vi "Main UI.vi"() -> ()   [LabVIEW 2016]
uses:
  Ctrls/Continuous Operations.ctl
  <vilib>/Utility/error.llb/DialogType.ctl
  HardWare/Ctrls/HardWare Gen _ DAQ Queue Names FGV Operations.ctl
  HardWare/Gantner/DAQ FGV Operations.ctl
  Architecture/Queue Management/ARC_Queue Create_Single.vi
  Architecture/Queue Management/ARC_Queue Valid.vi
  Architecture/Queue Management/ARC_Queue Remove Element.vi
  Ctrls/GlobeVaribles.vi
  Architecture/Queue Management/ARC_Queue Insert Element.vi
  Architecture/Queue Management/ARC_Queue Destroy_Single.vi
panel:
  in  "Tree":string(tree)
  in  "Stop":bool
  in  "Run":bool
  in  "Pause":bool
  out "notification":string
  out "变频器电压":sgl caption="Q1" format="%#.2f"
  out "变频器电流":sgl caption="Q2" format="%#.2f"
  out "变频器转速":sgl caption="Q3" format="%#.2f"
  out "变频器转矩":sgl caption="Q4" format="%#.2f"
  out "变频器加速时间":sgl caption="Q5" format="%#.2f"
  out "变频器减速时间":sgl caption="Q5" format="%#.2f"
  out "剩余时间":sgl caption="剩余时间:" format="%#.3g"
  out "设定时间":sgl caption="设定时间:" format="%#.3g"
  out "Error Report":string
  # "秒"
  # "秒"
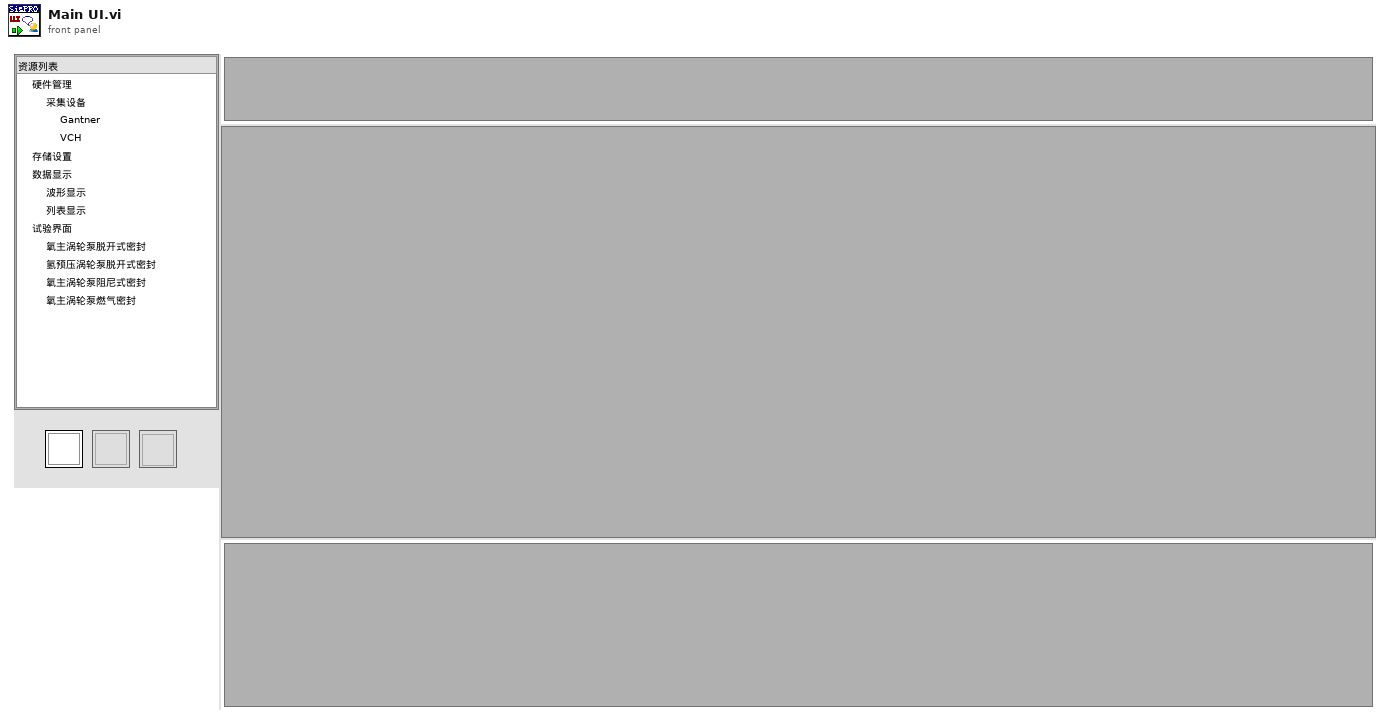
[diagram p1: front panel]
types:
  T1 = enum32{"Invalid", "Standard", "Closed", "Hidden", "Minimized", "Maximized"}
  T2 = enum16{"Obtain Notifier", "Send Notification", "Wait Notification", "Release Notifier"}
  T3 = typedef "Sys Paths.ctl" = cluster{"System Config":path, "User Archives":path, "Error Log":path, "DynaThreads":path, "TreePNG":path}
  T4 = typedef "User Login_Archives Data Structure.ctl" = cluster{"User Archives":cluster{"User Name":string, "Code":string, "Ability":enum16{"Administrator", "Operator"}, "Last Log Time":timestamp}[], "Current User":i32}
  T5 = cluster{"Error":errorcluster, "Exit":bool, "LocalQ":cluster{"LocalName":string, "LocalEvent":string, "LocalData":variant}, "Q-LowLevel":cluster{"Q-LowLevel Name":string, "Q-LowLevel Order":string, "Q-LowLevel Data":variant}, "Ref":cluster{"VIRef":refnum<vi>, "Tree":refnum<vi>}, "Threads":cluster{"Cfg":string, "Disp":string, "VCH":string, "Data":string, "SavePara":string}, "InsertUI":string, "Path":T3, "User Archives":T4, "FailedThreads":cluster{"ThreadName":string, "Fail":bool}[], "Buffers":cluster{"DataBuf":refnum<queue>}, "DevName":string}
  T6 = typedef "Continuous Operations.ctl" = enum16{"Writting", "Pause", "Stop"}
  T7 = typedef "HardWare Gen _ DAQ Queue Names FGV Operations.ctl" = enum16{"Initialize", "AddName", "ReadName"}
  T8 = typedef "DAQ FGV Operations.ctl" = enum16{"Search", "ReadCFG", "ReadVCH", "UpdateTempCFG", "DownloadCFG", "OpenCFG", "ImportPara", "Config", "Start", "Read", "Stop", "Clear"}
  T9 = typedef "DialogType.ctl" = u16
  T10 = cluster{"Run":refnum<vi>, "Pause":refnum<vi>, "Stop":refnum<vi>}
  T11 = cluster{"LocalName":string, "System Config":path, "DynaThreads":path, "DataBuf":refnum<queue>, "VIRef":refnum<vi>}
  T12 = cluster{"LocalName":string, "DataBuf":refnum<queue>}
  T13 = cluster{"LocalName":string, "System Config":path}
  T14 = typedef "LVRectTypeDef.ctl" = cluster{"Left":i16, "Top":i16, "Right":i16, "Bottom":i16}
  T15 = typedef "HardWare _ Module Configuration.ctl" = cluster{"ModuName":string, "ModuAlias":string, "ModuSN":string, "CHtype":string, "ParaNames[]":string[], "Paravalues[]":string[][]}
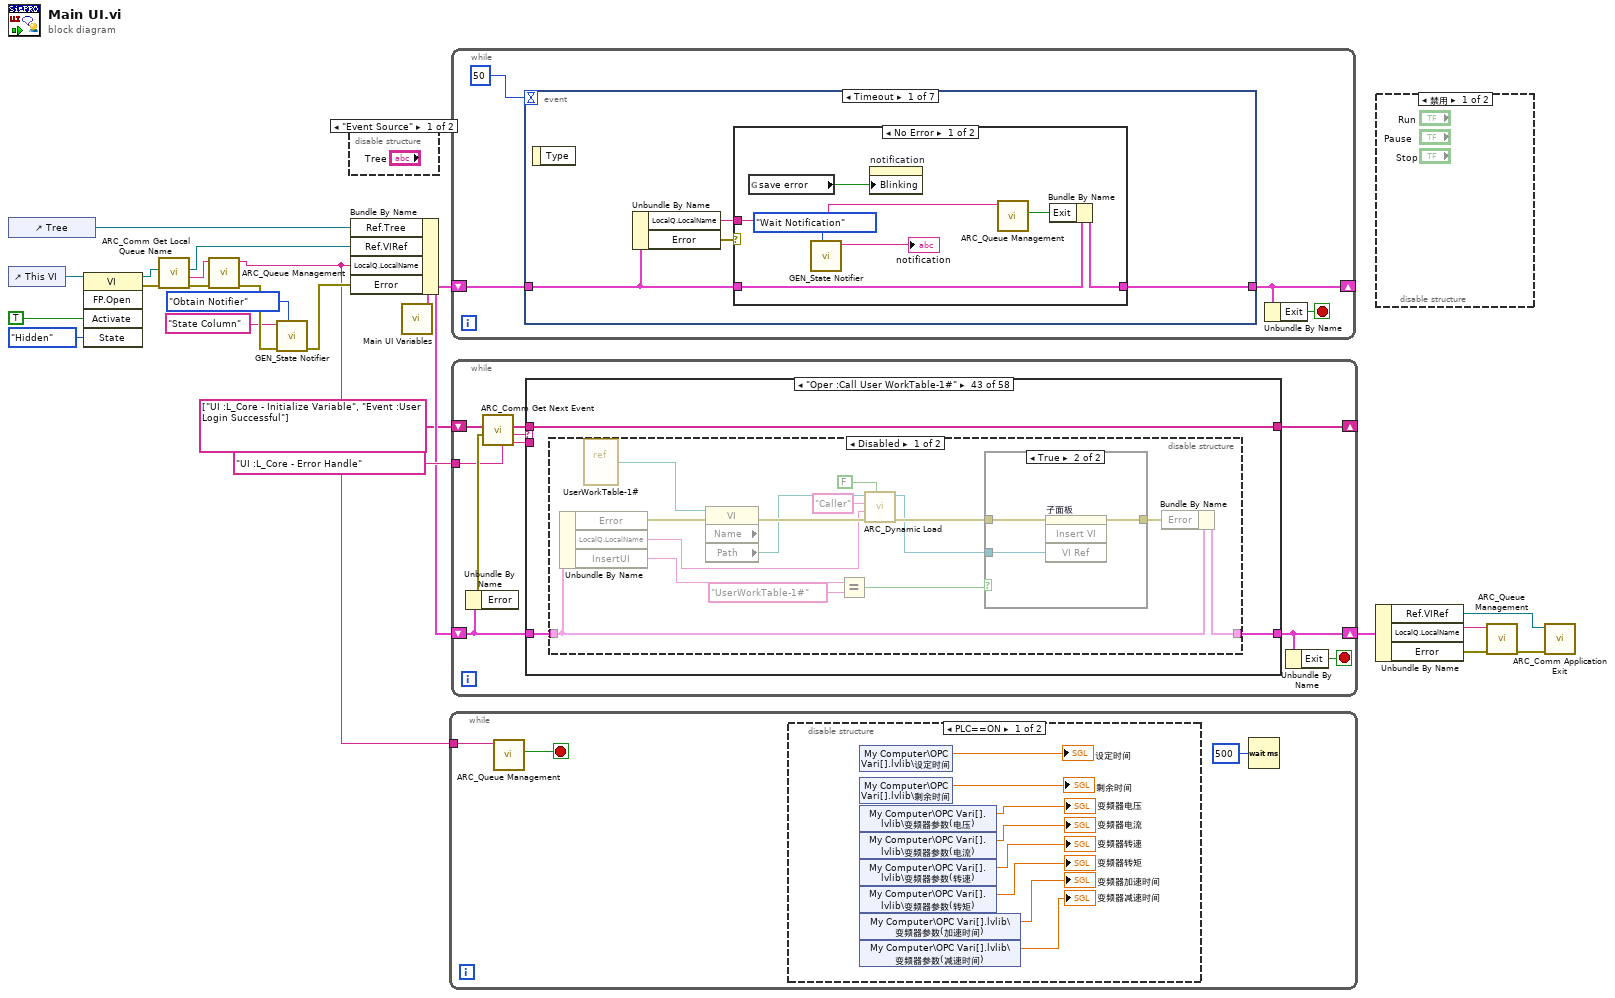
[diagram p0: block diagram]
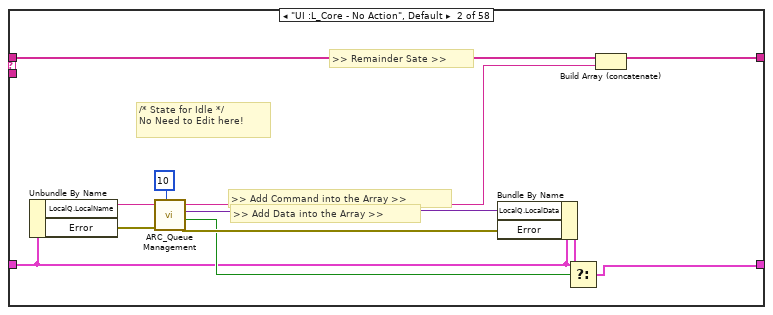
[diagram p6: hidden frame]
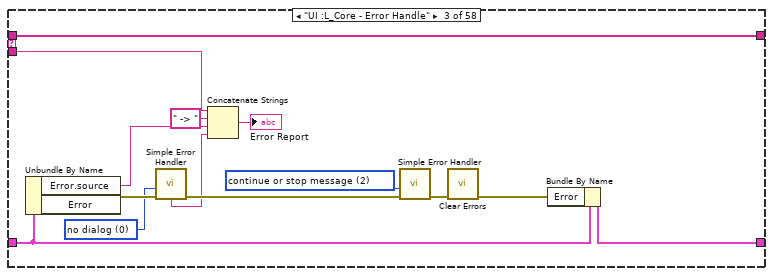
[diagram p7: hidden frame]
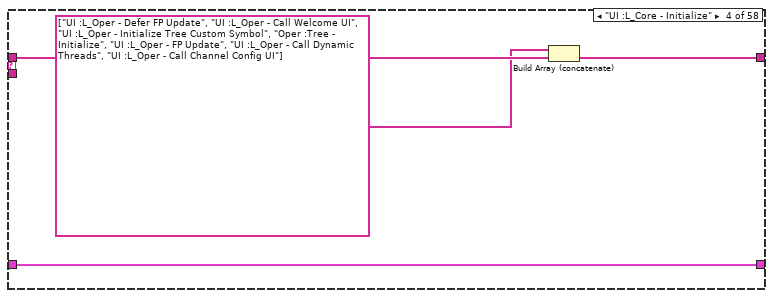
[diagram p8: hidden frame]
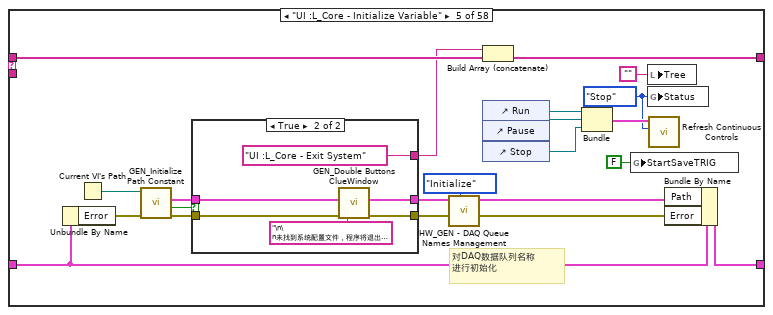
[diagram p9: hidden frame]
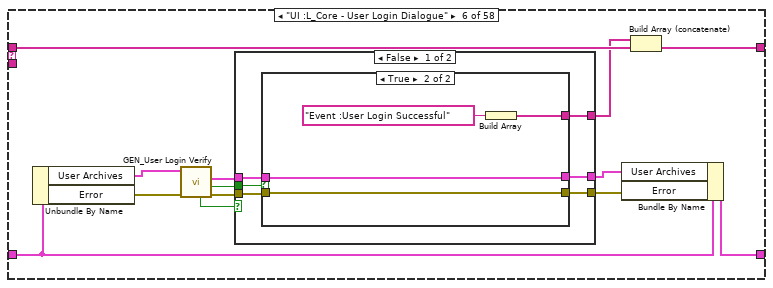
[diagram p11: hidden frame]
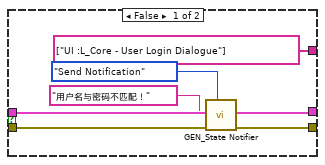
[diagram p12: hidden frame]
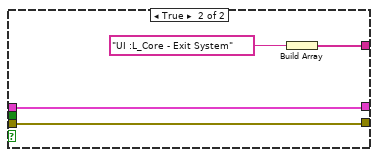
[diagram p13: hidden frame]
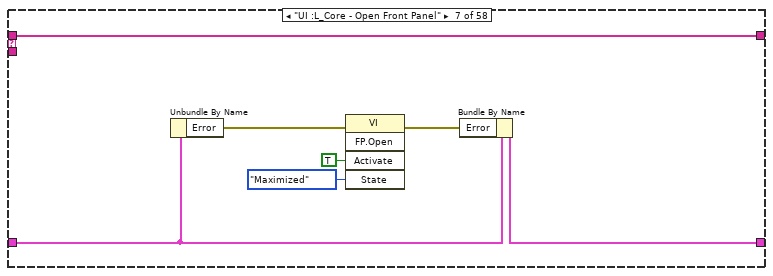
[diagram p14: hidden frame]
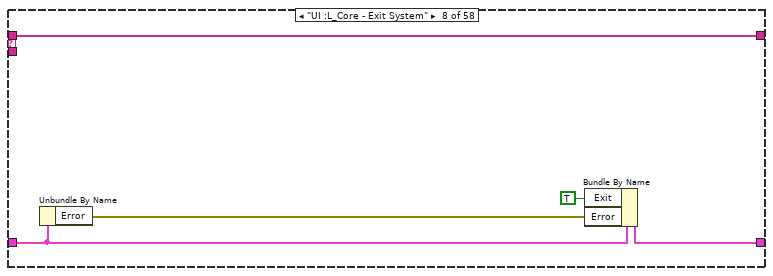
[diagram p15: hidden frame]
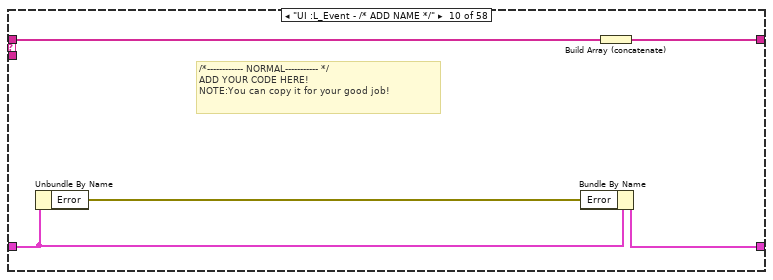
[diagram p17: hidden frame]
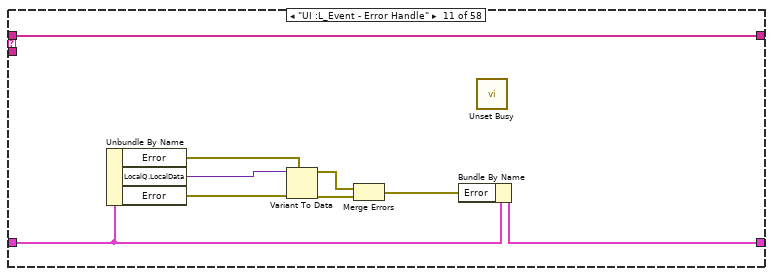
[diagram p18: hidden frame]
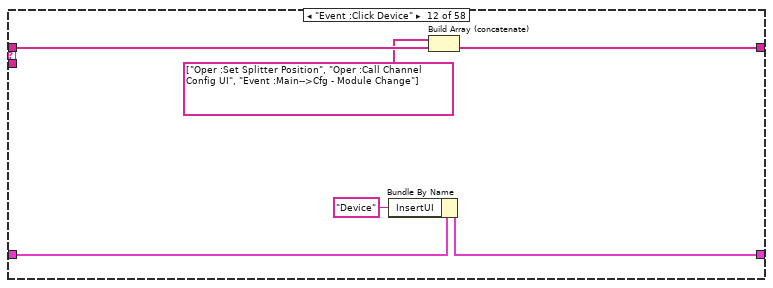
[diagram p19: hidden frame]
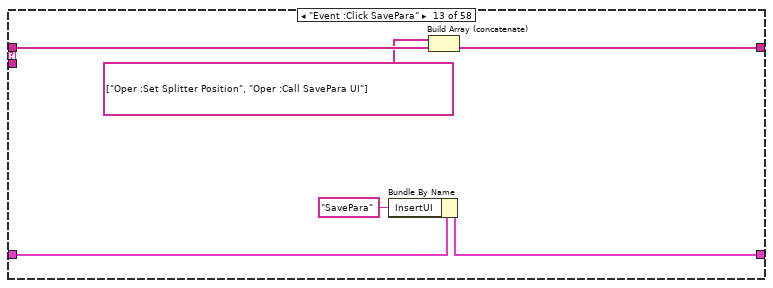
[diagram p20: hidden frame]
diagram:
  n1 = control-ref of="Tree"() -> (w15:refnum<vi>)
  n2 = control-ref of="This VI"() -> (w3:refnum<vi>)
  n3 = invoke class="VI" method="FP.Open"(reference=w3, "Activate"=TRUE ("激活？"), "State"=T1."Hidden" ("状态")) -> (reference out=w2:refnum<vi>, error out=w4:errorcluster)  [unwired: 2 in, 3 out]
  n4 = call "ARC_Comm Get Local Queue Name.vi"("error in"=w4, "VI Ref"=w2) -> ("error out"=w12:errorcluster, "VI  Name"=w14:string, "VI Ref out"=w13:refnum<vi>)  [unwired: 7 in]
  n5 = call-poly "ARC_Queue Management.vi"("error in"=w12, "Queue Name"=w14) -> ("error out"=w11:errorcluster, "Queue Name dup"=w1:string)  [unwired: 7 in, 1 out]
  n6 = call "GEN_State Notifier.vi"("Action Select"=T2."Obtain Notifier", "error in (no error)"=w11, "Notifier Name"="State Column") -> ("error out"=w10:errorcluster)  [unwired: 7 in, 1 out]
  n7 = disable-structure shown="\"Event Source\"" {
    frame condition #0 (active) {
    }
    frame condition #1 {
    }
  }
  n8 = call "Main UI Variables.vi"() -> ("Main UI.vi"=w16:T5)  [unwired: 11 in]
  n9 = Bundle By Name(cluster=w16, "Ref.Tree"=w15, "Ref.VIRef"=w13, "LocalQ.LocalName"=w1, "Error"=w10) -> (w20:T5)
  n10 = while {
    tunnel: w1 -> [w25]
    stop <- w24 stop-if-true
    n11 = call-poly "ARC_Queue Management.vi"("Queue Name(unamed)"=w25) -> ("Not Exist?"=w24:bool)  [unwired: 8 in, 2 out]
    n12 = disable-structure shown="PLC==ON" {
      frame condition #0 (active) {
        n13 = shared-variable "My Computer\\OPC Vari[].lvlib\\设定时间"() -> (→"设定时间":sgl)  [unwired: 1 in, 1 out]
        n14 = shared-variable "My Computer\\OPC Vari[].lvlib\\剩余时间"() -> (→"剩余时间":sgl)  [unwired: 1 in, 1 out]
        n15 = shared-variable "My Computer\\OPC Vari[].lvlib\\变频器参数(电压)"() -> (→"变频器电压":sgl)  [unwired: 1 in, 1 out]
        n16 = shared-variable "My Computer\\OPC Vari[].lvlib\\变频器参数(电流)"() -> (→"变频器电流":sgl)  [unwired: 1 in, 1 out]
        n17 = shared-variable "My Computer\\OPC Vari[].lvlib\\变频器参数(转速)"() -> (→"变频器转速":sgl)  [unwired: 1 in, 1 out]
        n18 = shared-variable "My Computer\\OPC Vari[].lvlib\\变频器参数(转矩)"() -> (→"变频器转矩":sgl)  [unwired: 1 in, 1 out]
        n19 = shared-variable "My Computer\\OPC Vari[].lvlib\\变频器参数(加速时间)"() -> (→"变频器加速时间":sgl)  [unwired: 1 in, 1 out]
        n20 = shared-variable "My Computer\\OPC Vari[].lvlib\\变频器参数(减速时间)"() -> (→"变频器减速时间":sgl)  [unwired: 1 in, 1 out]
      }
      frame condition #1 {
      }
    }
    n21 = Wait (ms)(milliseconds to wait=u32 500 ("等待时间（毫秒）")) -> ()  [unwired: 1 out]
  }
  n22 = while {
    shift-right: [w36] -> _
    shift-left: w20 -> [w37]
    stop <- w35 stop-if-true
    n23 = event shown="[0] Timeout" {
      selector: _ -> [_ _ _ _ _ _ _]
      dyn-events: _ -> [_ _ _ _ _ _ _]
      timeout: 50 -> [_ _ _ _ _ _ _]
      tunnel: w37 -> [w41 w61 w65 w79 w93 w113 w123]
      tunnel: [w42 w60 w64 w77 w92 w112 w122] -> w36
      event Timeout {
        n24 = event-data() -> ()  [unwired: 1 in, 1 out]
        n25 = Unbundle By Name(w41) -> ("LocalQ.LocalName"=w40:string, "Error"=w39:errorcluster)
        n26 = case shown="No Error" w39 {
          selector: w39 -> [_ w56]
          tunnel: [w49 w54] -> w42
          tunnel: w41 -> [w47 w55]
          tunnel: w40 -> [w46 w53]
          frame No Error {
            n27 = global read "GlobeVaribles.vi" "save error"() -> (w44:bool)
            n28 = call "GEN_State Notifier.vi"("Action Select"=T2."Wait Notification") -> ("Notification out"=→"notification":string)  [unwired: 9 in, 1 out]
            n29 = property on="notification" class="Str"("Blinking"=w44) -> ()  [unwired: 2 in, 2 out]
            n30 = call-poly "ARC_Queue Management.vi"("Queue Name(unamed)"=w46) -> ("Not Exist?"=w48:bool)  [unwired: 8 in, 2 out]
            n31 = Bundle By Name(cluster=w47, "Exit"=w48) -> (w49:T5)
          }
          frame Error {
            n32 = To Variant(anything=w56) -> (Variant=w51:variant)
            n33 = call "ARC_Queue Insert Single Messenges.vi"("Data"=w51, "Order"="UI :L_Event - Error Handle" ("Event"), "Queue Name"=w53) -> ("error out"=w50:errorcluster)  [unwired: 8 in]
            n34 = Bundle By Name(cluster=w55, "Error"=w50) -> (w54:T5)
          }
        }
      }
      event Panel Close? {
        n35 = event-data() -> ()  [unwired: 1 in, 1 out]
        n36 = Unbundle By Name(w61) -> ("LocalQ.LocalName"=w58:string, "Error"=w62:errorcluster)
        n37 = call-poly "ARC_Queue Management.vi"("error in (no error)"=w62, "Event"="UI :L_Event - Exit Event", "Queue Name(unamed)"=w58) -> ("error out"=w59:errorcluster)  [unwired: 7 in, 1 out]
        n38 = Bundle By Name(cluster=w61, "Error"=w59) -> (w60:T5)
        n39 = event-data("Discard?"=TRUE ("放弃？")) -> ()  [unwired: 1 in, 1 out]
      }
      event Panel Resize {
        n40 = event-data() -> ()  [unwired: 1 in, 1 out]
        n41 = Unbundle By Name(w65) -> ("LocalQ.LocalName"=w66:string, "Error"=w68:errorcluster)
        n42 = call-poly "ARC_Queue Management.vi"("error in (no error)"=w68, "Event"="Oper :Set Splitter Position", "Queue Name(unamed)"=w66) -> ("error out"=w67:errorcluster)  [unwired: 7 in, 1 out]
        n43 = Bundle By Name(cluster=w65, "Error"=w67) -> (w64:T5)
      }
      event "Tree": Value Change {
        n44 = event-data() -> ("CtlRef"=w80:refnum<vi>, "NewVal"=w70:string)  [unwired: 1 in]
        n45 = Unbundle By Name(w79) -> ("Error"=w78:errorcluster, "LocalQ.LocalName"=w72:string)
        n46 = call "Main Tree _ Click Event Pharse(tag).vi"("error in"=w78, "tag in"=w70, "Ref.Tree Ref"=w80) -> ("error out"=w75:errorcluster, "cmd?"=w76:bool, "LocalData"=w74:variant, "LocalEvent"=w73:string)  [unwired: 5 in]
        n47 = case shown="True" w76 {
          tunnel: w75 -> [w81 w87]
          tunnel: w74 -> [_ w86]
          tunnel: w73 -> [_ w84]
          tunnel: w72 -> [_ w85]
          tunnel: [w81 w83] -> w71
          frame False {
          }
          frame True {
            n48 = call-poly "ARC_Queue Management.vi"("Time out(-1)_queue in"=20, "error in (no error)"=w87, "Data"=w86, "Event"=w84, "Queue Name(unamed)"=w85) -> ("error out"=w83:errorcluster)  [unwired: 5 in, 1 out]
          }
        }
        n49 = Bundle By Name(cluster=w79, "Error"=w71) -> (w77:T5)
      }
      event "Run": Value Change {
        n50 = event-data() -> ("CtlRef"=w94:refnum<vi>)  [unwired: 1 in]
        n51 = Unbundle By Name(w93) -> ("LocalQ.LocalName"=w91:string, "Error"=w95:errorcluster)
        n52 = invoke class="Bool" method="Reinit To Default"(reference=w94, error in=w95) -> (error out=w96:errorcluster)  [unwired: 1 in, 2 out]
        n53 = global read "GlobeVaribles.vi" "Status"() -> (w90:T6)
        n54 = case shown="\"Stop\"" w90 {
          tunnel: w96 -> [w100 w102 w107]
          tunnel: [w100 w102 w105] -> w89
          tunnel: w91 -> [_ _ w103]
          frame "Writting" {
          }
          frame "Pause", Default {
            n55 = global write "GlobeVaribles.vi" "Status"(Continuous_Operations."Writting" ("Status")) -> ()
          }
          frame "Stop" {
            n56 = call-poly "ARC_Queue Management.vi"("Time out(-1)_queue in"=50, "error in (no error)"=w107, "Event"="Event :Start Save", "Queue Name(unamed)"=w103) -> ("error out"=w105:errorcluster)  [unwired: 6 in, 1 out]
          }
        }
        n57 = flat-sequence {
          tunnel: w89 -> [w98]
          tunnel: [w97] -> w88
          frame #0 {
            n58 = call "Refresh Continuous Controls.vi"("error in"=w98, "Cmd"=Continuous_Operations."Writting") -> ("error out"=w97:errorcluster)  [unwired: 9 in]
          }
        }
        n59 = Bundle By Name(cluster=w93, "Error"=w88) -> (w92:T5)
      }
      event "Pause": Value Change {
        w108 = Continuous_Operations."Pause" ("Cmd")
        n60 = event-data() -> ("CtlRef"=w114:refnum<vi>)  [unwired: 1 in]
        n61 = Unbundle By Name(w113) -> ("LocalQ.LocalName"=w109:string, "Error"=w115:errorcluster)
        n62 = invoke class="Bool" method="Reinit To Default"(reference=w114, error in=w115) -> (error out=w117:errorcluster)  [unwired: 1 in, 2 out]
        n63 = call-poly "ARC_Queue Management.vi"("Time out(-1)_queue in"=50, "error in (no error)"=w117, "Event"="Event :Pause Save", "Queue Name(unamed)"=w109) -> ("error out"=w111:errorcluster)  [unwired: 6 in, 1 out]
        n64 = call "Refresh Continuous Controls.vi"("Cmd"=w108) -> ()  [unwired: 10 in, 1 out]
        n65 = global write "GlobeVaribles.vi" "Status"(w108) -> ()
        n66 = Bundle By Name(cluster=w113, "Error"=w111) -> (w112:T5)
      }
      event "Stop": Value Change {
        w118 = Continuous_Operations."Stop" ("Cmd")
        n67 = event-data() -> ("CtlRef"=w124:refnum<vi>)  [unwired: 1 in]
        n68 = Unbundle By Name(w123) -> ("LocalQ.LocalName"=w119:string, "Error"=w125:errorcluster)
        n69 = invoke class="Bool" method="Reinit To Default"(reference=w124, error in=w125) -> (error out=w127:errorcluster)  [unwired: 1 in, 2 out]
        n70 = call-poly "ARC_Queue Management.vi"("Time out(-1)_queue in"=50, "error in (no error)"=w127, "Event"="Event :Stop Save", "Queue Name(unamed)"=w119) -> ("error out"=w121:errorcluster)  [unwired: 6 in, 1 out]
        n71 = call "Refresh Continuous Controls.vi"("Cmd"=w118) -> ()  [unwired: 10 in, 1 out]
        n72 = global write "GlobeVaribles.vi" "Status"(w118) -> ()
        n73 = Bundle By Name(cluster=w123, "Error"=w121) -> (w122:T5)
      }
    }
    n74 = Unbundle By Name(w36) -> ("Exit"=w35:bool)
  }
  n75 = while {
    shift-right: [w131] -> w17
    shift-left: w20 -> [w133]
    shift-right: [w134] -> _
    shift-left: string[] ["UI :L_Core - Initialize Variable", "Event :User Login Successful"] ("event queue out") -> [w137]
    tunnel: "UI :L_Core - Error Handle" ("Error Handle") -> [w129]
    stop <- w130 stop-if-true
    n76 = Unbundle By Name(w133) -> ("Error"=w132:errorcluster)
    n77 = call "ARC_Comm Get Next Event.vi"("Error Handle"=w129, "error in (no error)"=w132, "event queue in"=w137) -> ("prev event"=w128:string, "next event"=w136:string, "event queue out"=w135:string[])  [unwired: 3 in]
    n78 = case shown="\"Oper :Call User WorkTable-1#\"" w136 {
      selector: w136 -> [_ _ _ _ _ _ _ _ _ _ _ _ _ _ _ _ _ _ _ _ _ _ _ _ _ w319 w328 w337 w346 w355 w366 w375 w386 _ _ _ _ _ _ _ _ _ _ _ _ _ _ _ _ _ _ _ _ _ _ _ _ _]
      tunnel: w133 -> [w138 w142 w163 w166 w186 w209 w232 w239 w243 w248 w251 w263 w269 w275 w281 w287 w293 w295 w297 w301 w303 w307 w309 w313 w317 w326 w335 w344 w353 w362 w372 w381 w392 w394 w401 w424 w465 w506 w547 w576 w604 w617 w628 w659 w681 w702 w725 w731 w735 w746 w757 w759 w770 w782 w790 w799 w801 w803]
      tunnel: w135 -> [w139 w148 w165 w169 w190 w210 w237 w242 w244 w246 w258 w264 w270 w276 w282 w288 w291 w296 w298 w302 w306 w308 w312 w316 w318 w327 w336 w345 w354 w363 w373 w382 w393 w395 w404 w429 w470 w511 w552 w583 w610 w622 w629 w665 w682 w703 w726 w732 w743 w754 w758 w761 w771 w783 w791 w800 w802 w811]
      tunnel: [w139 w147 w165 w168 w183 w202 w237 w242 w244 w245 w258 w262 w268 w274 w280 w286 w290 w296 w298 w300 w305 w308 w311 w315 w318 w324 w333 w342 w351 w360 w373 w382 w393 w395 w399 w429 w470 w511 w552 w583 w610 w622 w629 w665 w677 w703 w726 w732 w743 w754 w758 w761 w771 w779 w791 w800 w802 w811] -> w134
      tunnel: [w138 w140 w164 w166 w188 w200 w231 w240 w243 w247 w250 w260 w266 w272 w278 w284 w292 w295 w297 w301 w303 w307 w309 w313 w317 w325 w334 w343 w352 w361 w368 w377 w388 w394 w397 w423 w464 w505 w546 w575 w603 w616 w627 w658 w675 w695 w724 w730 w734 w745 w757 w759 w767 w780 w786 w794 w801 w810] -> w131
      tunnel: w128 -> [_ _ w153 _ _ _ _ _ _ _ _ _ _ _ _ _ _ _ _ _ _ _ _ _ _ _ _ _ _ _ _ _ _ _ _ _ _ _ _ _ _ _ _ _ _ _ _ _ _ _ _ _ _ _ _ _ _ _]
      frame "----------Core Status----------" {
      }
      frame "UI :L_Core - No Action", Default {
        # "/* State for Idle */\nNo Need to Edit here!"
        # ">> Add Data into the Array >>"
        # ">> Add Command into the Array >>"
        # ">> Remainder Sate >>"
        n79 = Unbundle By Name(w142) -> ("LocalQ.LocalName"=w145:string, "Error"=w149:errorcluster)
        n80 = call-poly "ARC_Queue Management.vi"("Time out(-1)_queue out"=10, "error in (no error)"=w149, "Queue Name(unamed)"=w145) -> ("error out"=w151:errorcluster, "timed out"=w143:bool, "Data"=w150:variant, "Event"=w146:string)  [unwired: 5 in]
        n81 = Bundle By Name(cluster=w142, "LocalQ.LocalData"=w150, "Error"=w151) -> (w141:T5)
        n82 = Select(t=w142, s=w143, f=w141) -> (s? t:f=w140:T5)
        n83 = Build Array (concatenate)(w148, w146) -> (w147:string[])
      }
      frame "UI :L_Core - Error Handle" {
        w152 = T9 0 items=["no dialog", "OK message", "continue or stop message", "OK message + warnings", "continue/stop + warnings"] ("type of dialog (OK msg:1)")
        w160 = T9 2 items=["no dialog", "OK message", "continue or stop message", "OK message + warnings", "continue/stop + warnings"] ("type of dialog (OK msg:1)")
        n84 = Unbundle By Name(w163) -> ("Error.source"=w154:string, "Error"=w157:errorcluster)
        n85 = call <vilib>:"Simple Error Handler.vi"("type of dialog (OK msg:1)"=w152, "error in (no error)"=w157) -> ("error out"=w156:errorcluster, "message"=w155:string)  [unwired: 3 in, 3 out]
        n86 = Concatenate Strings(w153, " -> " ("字符串"), w154, w155) -> (→"Error Report":string)
        n87 = call <vilib>:"Simple Error Handler.vi"("type of dialog (OK msg:1)"=w160, "error in (no error)"=w156) -> ("error out"=w162:errorcluster)  [unwired: 3 in, 4 out]
        n88 = call <vilib>:"Clear Errors.vi"("error in (no error)"=w162) -> ("error out"=w161:errorcluster)  [unwired: 5 in, 1 out]
        n89 = Bundle By Name(cluster=w163, "Error"=w161) -> (w164:T5)
      }
      frame "UI :L_Core - Initialize" {
        n90 = Build Array (concatenate)(string[] ["UI :L_Oper - Defer FP Update", "UI :L_Oper - Call Welcome UI", "UI :L_Oper - Initialize Tree Custom Symbol", "Oper :Tree - Initialize", "UI :L_Oper - FP Update", "UI :L_Oper - Call Dynamic Threads", "UI :L_Oper - Call Channel Config UI"], w169) -> (w168:string[])
      }
      frame "UI :L_Core - Initialize Variable" {
        w174 = Continuous_Operations."Stop" ("Status")
        # "对DAQ数据队列名称\n进行初始化"
        n91 = Unbundle By Name(w186) -> ("Error"=w185:errorcluster)
        n92 = Current VI's Path() -> (path=w187:path)
        n93 = call "GEN_Initialize Path Constant.vi"("error in"=w185, "Path in"=w187) -> ("error out"=w184:errorcluster, "File not exists?"=w181:bool, "Path Constant"=w180:T3)  [unwired: 6 in, 1 out]
        n94 = case shown="True" w181 {
          tunnel: w184 -> [w192 w195]
          tunnel: [w192 w194] -> w178
          tunnel: w180 -> [w191 w197]
          tunnel: [w191 w197] -> w179
          tunnel: [_ "UI :L_Core - Exit System"] -> w182
          frame False {
          }
          frame True {
            n95 = call "GEN_Double Buttons ClueWindow.vi"("error in (no error)"=w195, "Content Input"="\n\n未找到系统配置文件，程序将退出！" ("消息")) -> ("error out"=w194:errorcluster)  [unwired: 7 in, 2 out]
          }
        }
        n96 = call "HW_GEN - DAQ Queue Names Management.vi"("Oper."=HardWare_Gen___DAQ_Queue_Names_FGV_Operations."Initialize", "error in"=w178) -> ("error out"=w177:errorcluster)  [unwired: 8 in, 1 out]
        n97 = Build Array (concatenate)(w182, w190) -> (w183:string[])
        n98 = control-ref of="Run"() -> (w173:refnum<vi>)
        n99 = control-ref of="Pause"() -> (w172:refnum<vi>)
        n100 = control-ref of="Stop"() -> (w171:refnum<vi>)
        n101 = Bundle("Run"=w173, "Pause"=w172, "Stop"=w171) -> (w175:T10)  [unwired: 1 in]
        n102 = global write "GlobeVaribles.vi" "StartSaveTRIG"(FALSE ("StartSaveTRIG")) -> ()
        n103 = local write "Tree"("") -> ()
        n104 = global write "GlobeVaribles.vi" "Status"(w174) -> ()
        n105 = call "Refresh Continuous Controls.vi"("Cmd"=w174, "Ctrls"=w175) -> ()  [unwired: 9 in, 1 out]
        n106 = Bundle By Name(cluster=w186, "Path"=w179, "Error"=w177) -> (w188:T5)
      }
      frame "UI :L_Core - User Login Dialogue" {
        n107 = Unbundle By Name(w209) -> ("User Archives"=w208:T4, "Error"=w207:errorcluster)
        n108 = call "GEN_User Login Verify.vi"("error in"=w207, "User Archives"=w208) -> ("error out"=w206:errorcluster, "User Exist?"=w203:bool, "User Archives out"=w204:T4, "Cancel?"=w205:bool)  [unwired: 6 in]
        n109 = case shown="False" w205 {
          tunnel: w203 -> [w216 _]
          tunnel: w206 -> [w215 w228]
          tunnel: w204 -> [w214 w227]
          tunnel: [w213 w228] -> w199
          tunnel: [w212 w227] -> w198
          tunnel: [w211 w229] -> w201
          frame False {
            n110 = case shown="True" w216 {
              tunnel: w215 -> [w218 w226]
              tunnel: w214 -> [w222 w225]
              tunnel: [w222 w225] -> w212
              tunnel: [w219 w226] -> w213
              tunnel: [string[] ["UI :L_Core - User Login Dialogue"] w223] -> w211
              frame False {
                n111 = call "GEN_State Notifier.vi"("Action Select"=T2."Send Notification", "error in (no error)"=w218, "Notification"="用户名与密码不匹配！") -> ("error out"=w219:errorcluster)  [unwired: 7 in, 1 out]
              }
              frame True {
                n112 = Build Array("Event :User Login Successful") -> (w223:string[])
              }
            }
          }
          frame True {
            n113 = Build Array("UI :L_Core - Exit System") -> (w229:string[])
          }
        }
        n114 = Bundle By Name(cluster=w209, "User Archives"=w198, "Error"=w199) -> (w200:T5)
        n115 = Build Array (concatenate)(w201, w210) -> (w202:string[])
      }
      frame "UI :L_Core - Open Front Panel" {
        n116 = Unbundle By Name(w232) -> ("Error"=w235:errorcluster)
        n117 = invoke class="VI" method="FP.Open"(error in=w235, "Activate"=TRUE ("激活？"), "State"=T1."Maximized" ("状态")) -> (error out=w236:errorcluster)  [unwired: 2 in, 4 out]
        n118 = Bundle By Name(cluster=w232, "Error"=w236) -> (w231:T5)
      }
      frame "UI :L_Core - Exit System" {
        n119 = Unbundle By Name(w239) -> ("Error"=w241:errorcluster)
        n120 = Bundle By Name(cluster=w239, "Exit"=TRUE, "Error"=w241) -> (w240:T5)
      }
      frame "----------Events----------" {
        # ">> Notes: 此处分支主要用于响应事件结构，考虑多个事件的合并，可在此处执行代码后进行界面刷新；<<"
      }
      frame "UI :L_Event - /* ADD NAME */" {
        # "/*------------ NORMAL----------- */\nADD YOUR CODE HERE!\nNOTE:You can copy it for your good job!"
        n121 = Unbundle By Name(w248) -> ("Error"=w249:errorcluster)
        n122 = Bundle By Name(cluster=w248, "Error"=w249) -> (w247:T5)
        n123 = Build Array (concatenate)(w246) -> (w245:string[])
      }
      frame "UI :L_Event - Error Handle" {
        n124 = Unbundle By Name(w251) -> ("Error"=w255:errorcluster, "LocalQ.LocalData"=w256:variant, "Error"=w257:errorcluster)
        n125 = Variant To Data(error in=w257, type=w255, Variant=w256) -> (data=w254:errorcluster, error out=w252:errorcluster)
        n126 = Merge Errors(w254, w252) -> (w253:errorcluster)
        n127 = Bundle By Name(cluster=w251, "Error"=w253) -> (w250:T5)
        n128 = call <vilib>:"Unset Busy.vi"() -> ()  [unwired: 11 in, 1 out]
      }
      frame "Event :Click Device" {
        n129 = Bundle By Name(cluster=w263, "InsertUI"="Device") -> (w260:T5)
        n130 = Build Array (concatenate)(string[] ["Oper :Set Splitter Position", "Oper :Call Channel Config UI", "Event :Main-->Cfg - Module Change"] ("数组"), w264) -> (w262:string[])
      }
      frame "Event :Click SavePara" {
        n131 = Bundle By Name(cluster=w269, "InsertUI"="SavePara") -> (w266:T5)
        n132 = Build Array (concatenate)(string[] ["Oper :Set Splitter Position", "Oper :Call SavePara UI"] ("数组"), w270) -> (w268:string[])
      }
      frame "Event :Click Graph" {
        # "//单击波形图显示界面"
        n133 = Bundle By Name(cluster=w275, "InsertUI"="Q_Disp") -> (w272:T5)
        n134 = Build Array (concatenate)(string[] ["Oper :Set Splitter Position", "Oper :Call Display Graph", "Event :Main-->Disp - Graph UI"] ("数组"), w276) -> (w274:string[])
      }
      frame "Event :Click List" {
        # "//单击列表显示界面"
        n135 = Bundle By Name(cluster=w281, "InsertUI"="Q_Disp") -> (w278:T5)
        n136 = Build Array (concatenate)(string[] ["Oper :Set Splitter Position", "Oper :Call Display Graph", "Event :Main-->Disp - List UI"] ("数组"), w282) -> (w280:string[])
      }
      frame "Event :Click UserWorkTable-1#" {
        n137 = Bundle By Name(cluster=w287, "InsertUI"="UserWorkTable-1#") -> (w284:T5)
        n138 = Build Array (concatenate)(string[] ["Oper :Set Splitter Position", "Oper :Call User WorkTable-1#", "Event :Main-->Disp - List UI"] ("数组"), w288) -> (w286:string[])
      }
      frame "UI :L_Event - Exit Event" {
        n139 = Unbundle By Name(w293) -> ("Error"=w294:errorcluster)
        n140 = Bundle By Name(cluster=w293, "Error"=w294) -> (w292:T5)
        n141 = Build Array (concatenate)(w291, string[] ["UI :L_Core - Exit System"] ("数组")) -> (w290:string[])
      }
      frame "----------events from other threads----------" {
      }
      frame "Event :Error Handle" {
      }
      frame "Event :User Login Successful" {
        n142 = Build Array (concatenate)(string[] ["UI :L_Oper - Defer FP Update", "UI :L_Oper - Set Mouse Busy", "UI :L_Oper - Initialize Tree Custom Symbol", "Oper :Tree - Initialize", "Oper :Set Splitter Position", "Oper :Set User Group Menus", "UI :L_Oper - FP Update", "Oper :Create Buffers", "Oper :Call Dynamic Threads", "Oper :Scan for Devices", "UI :L_Oper - Set Mouse Free"], w302) -> (w300:string[])
      }
      frame "Event :Cfg-->M - Update ChanPara" {
        # "//接收配置线程发送过来的设备参数信息修改命令"
        n143 = Build Array (concatenate)(string[] ["Event :Main-->Disp - Update Channel Para", "Event :Main-->Data - Update Channel Para"] ("数组"), w306) -> (w305:string[])
      }
      frame "Event :Cfg-->M - Unbusy Mouse" {
        n144 = call <vilib>:"Unset Busy.vi"() -> ()  [unwired: 11 in, 1 out]
      }
      frame "Event :Start Save" {
        # "主线程收到显示线程的命令，启动连续存储；\n主线程向数据线程发送命令；"
        n145 = Build Array (concatenate)("Event :Main-->Data - Start Save", w312) -> (w311:string[])
      }
      frame "Event :Stop Save" {
        # "主线程收到显示线程的命令，停止连续存储；\n主线程向数据线程发送命令；"
        n146 = Build Array (concatenate)("Event :Main-->Data - Stop Save", w316) -> (w315:string[])
      }
      frame "---------------send to other threads--------------" {
      }
      frame "Event :Main-->Cfg - Module Change" {
        # "//单击tree上某模块名称后，向配置线程发送选择的模块信息"
        n147 = Unbundle By Name(w326) -> ("Threads.Cfg"=w322:string, "LocalQ.LocalData"=w320:variant, "Error"=w321:errorcluster)
        n148 = Bundle By Name(cluster=w326, "Q-LowLevel.Q-LowLevel Order"=w319, "Q-LowLevel.Q-LowLevel Name"=w322, "Q-LowLevel.Q-LowLevel Data"=w320, "Error"=w321) -> (w325:T5)
        n149 = Build Array (concatenate)("Oper :Send To LowLevel" ("Error Handle"), w327) -> (w324:string[])
        n150 = call <vilib>:"Set Busy.vi"() -> ()  [unwired: 10 in, 2 out]
      }
      frame "Event :Main-->Cfg - Start DAQ" {
        # "//单击tree上某模块名称后，向配置线程发送选择的模块信息"
        n151 = Unbundle By Name(w335) -> ("Threads.Cfg"=w331:string, "LocalQ.LocalData"=w329:variant, "Error"=w330:errorcluster)
        n152 = Bundle By Name(cluster=w335, "Q-LowLevel.Q-LowLevel Order"=w328, "Q-LowLevel.Q-LowLevel Name"=w331, "Q-LowLevel.Q-LowLevel Data"=w329, "Error"=w330) -> (w334:T5)
        n153 = Build Array (concatenate)("Oper :Send To LowLevel" ("Error Handle"), w336) -> (w333:string[])
      }
      frame "Event :Main-->Disp - Update Channel Para" {
        n154 = Unbundle By Name(w344) -> ("Threads.Disp"=w340:string, "LocalQ.LocalData"=w338:variant, "Error"=w339:errorcluster)
        n155 = Bundle By Name(cluster=w344, "Q-LowLevel.Q-LowLevel Order"=w337, "Q-LowLevel.Q-LowLevel Name"=w340, "Q-LowLevel.Q-LowLevel Data"=w338, "Error"=w339) -> (w343:T5)
        n156 = Build Array (concatenate)("Oper :Send To LowLevel" ("Error Handle"), w345) -> (w342:string[])
      }
      frame "Event :Main-->Disp - Graph UI" {
        n157 = Unbundle By Name(w353) -> ("Threads.Disp"=w349:string, "LocalQ.LocalData"=w347:variant, "Error"=w348:errorcluster)
        n158 = Bundle By Name(cluster=w353, "Q-LowLevel.Q-LowLevel Order"=w346, "Q-LowLevel.Q-LowLevel Name"=w349, "Q-LowLevel.Q-LowLevel Data"=w347, "Error"=w348) -> (w352:T5)
        n159 = Build Array (concatenate)("Oper :Send To LowLevel" ("Error Handle"), w354) -> (w351:string[])
      }
      frame "Event :Main-->Disp - List UI" {
        n160 = Unbundle By Name(w362) -> ("Threads.Disp"=w358:string, "LocalQ.LocalData"=w356:variant, "Error"=w357:errorcluster)
        n161 = Bundle By Name(cluster=w362, "Q-LowLevel.Q-LowLevel Order"=w355, "Q-LowLevel.Q-LowLevel Name"=w358, "Q-LowLevel.Q-LowLevel Data"=w356, "Error"=w357) -> (w361:T5)
        n162 = Build Array (concatenate)("Oper :Send To LowLevel" ("Error Handle"), w363) -> (w360:string[])
      }
      frame "Event :Main-->Data - Start Save" {
        # "给启动存储的触发信号\n让DAQ线程建立时间通道信息"
        # "主线程收到显示线程的命令，启动连续存储；\n主线程向数据线程发送命令；"
        n163 = Unbundle By Name(w372) -> ("Threads.Data"=w370:string, "Error"=w371:errorcluster)
        n164 = call-poly "ARC_Queue Management.vi"("Time out(-1)_queue in"=50, "error in (no error)"=w371, "Event"=w366, "Queue Name(unamed)"=w370) -> ("error out"=w367:errorcluster)  [unwired: 6 in, 1 out]
        n165 = global read "GlobeVaribles.vi" "Status"() -> (w365:T6)
        n166 = case shown="\"Stop\"" w365 {
          tunnel: [_ TRUE ("StartSave")] -> w364
          frame "Writting", Default {
          }
          frame "Stop" {
          }
        }
        n167 = Bundle By Name(cluster=w372, "Error"=w367) -> (w368:T5)
        n168 = global write "GlobeVaribles.vi" "StartSaveTRIG"(w364) -> ()
      }
      frame "Event :Main-->Data - Stop Save" {
        # "主线程收到显示线程的命令，启动连续存储；\n主线程向数据线程发送命令；"
        n169 = Unbundle By Name(w381) -> ("Threads.Data"=w379:string, "Error"=w380:errorcluster)
        n170 = call-poly "ARC_Queue Management.vi"("Time out(-1)_queue in"=50, "error in (no error)"=w380, "Event"=w375, "Queue Name(unamed)"=w379) -> ("error out"=w376:errorcluster)  [unwired: 6 in, 1 out]
        n171 = Bundle By Name(cluster=w381, "Error"=w376) -> (w377:T5)
      }
      frame "Event :Main-->Data - Update Channel Para" {
        # "向数据线程发送更新通道参数命令"
        n172 = Unbundle By Name(w392) -> ("Threads.Data"=w390:string, "DevName"=w385:string, "LocalQ.LocalData"=w384:variant, "Error"=w391:errorcluster)
        n173 = Bundle("DevName"=w385, "LocalData"=w384) -> (w383:cluster{"DevName":string, "LocalData":variant})  [unwired: 1 in]
        n174 = call-poly "ARC_Queue Management.vi"("Time out(-1)_queue in"=50, "error in (no error)"=w391, "Data"=w383, "Event"=w386, "Queue Name(unamed)"=w390) -> ("error out"=w387:errorcluster)  [unwired: 5 in, 1 out]
        n175 = Bundle By Name(cluster=w392, "Error"=w387) -> (w388:T5)
      }
      frame "----------Operations----------" {
        # ">> Notes: 此处分支主要用于数据结构相关操作，并考虑复用；<<"
      }
      frame "Oper :Call Dynamic Threads" {
        n176 = Unbundle By Name(w401) -> ("Error"=w400:errorcluster)
        n177 = call "GEN_State Notifier.vi"("Action Select"=T2."Send Notification", "error in (no error)"=w400, "Notification"="正在加载动态模块...") -> ("error out"=w396:errorcluster)  [unwired: 7 in, 1 out]
        n178 = Build Array (concatenate)(string[] ["Oper :Call Error Handle", "Oper :Call Welcome UI", "UI :L_Core - Open Front Panel", "Oper :Call Channel Config UI", "Oper :Call Display Graph", "Oper :Call Data Thread", "Oper :Call SavePara UI", "Oper :Call OPC Read Bool UI", "Oper :Call DAQ Mean Data UI", "Oper :Call User WorkTable-1#", "Oper :Thread Loaded Fail"] ("数组"), w404) -> (w399:string[])
        n179 = Bundle By Name(cluster=w401, "Error"=w396) -> (w397:T5)
      }
      frame "Oper :Call Channel Config UI" {
        w408 = FALSE ("open front panel? (T)")
        n180 = vi-ref "HardWare_Phsical Channels Config_Gantner.vi"() -> (w406:refnum<vi>)
        n181 = Unbundle By Name(w424) -> ("FailedThreads"=w413:cluster{"ThreadName":string, "Fail":bool}[], "Error"=w426:errorcluster, "LocalQ.LocalName"=w422:string, "Path.System Config"=w418:path, "Path.DynaThreads"=w417:path, "Buffers.DataBuf"=w407:refnum<queue>, "Ref.VIRef"=w405:refnum<vi>, "InsertUI"=w421:string)
        n182 = property class="VI"(reference=w406, error in=w426) -> (reference out=w411:refnum<vi>, error out=w427:errorcluster, "Name"=w410:string, "Path"=w425:path)
        n183 = Bundle("LocalName"=w422, "System Config"=w418, "DynaThreads"=w417, "DataBuf"=w407, "VIRef"=w405) -> (w419:T11)  [unwired: 1 in]
        n184 = call "ARC_Dynamic Call_Single.vi"("command queue name"=w410, "open front panel? (T)"=w408, "error in (no error)"=w427, "parameter else"=w419, "control name"="Parameter", "vi path"=w425) -> ("error out"=w416:errorcluster, "call failed"=w414:bool)  [unwired: 3 in, 1 out]
        n185 = Equal?(x=w421, y="Device" ("control name")) -> (x = y?=w409:bool)
        n186 = case shown="False" w414 {
          selector: w414 -> [_ w449]
          tunnel: w416 -> [w433 w447]
          tunnel: w413 -> [w435 w450]
          tunnel: [w435 w448] -> w412
          tunnel: [w434 w447] -> w415
          tunnel: w409 -> [w432 _]
          tunnel: w411 -> [w431 _]
          tunnel: w410 -> [_ w446]
          tunnel: w408 -> [w430 _]
          frame False {
            n187 = case shown="True" w432 {
              tunnel: [w436 w440] -> w434
              tunnel: w431 -> [_ w439]
              tunnel: w433 -> [w436 w438]
              tunnel: w430 -> [_ w437]
              frame False {
              }
              frame True {
                n188 = case shown="False" w437 {
                  tunnel: [w443 w444] -> w440
                  tunnel: w439 -> [w442 _]
                  tunnel: w438 -> [w441 w444]
                  frame False {
                    n189 = invoke on="子面板" class="SubPnl" method="Insert VI"(error in=w441, "VI Ref"=w442) -> (error out=w443:errorcluster)  [unwired: 2 in, 3 out]
                  }
                  frame True {
                  }
                }
              }
            }
          }
          frame True {
            n190 = Bundle("Name"=w446, w449) -> (w445:cluster{"Name":string, bool})  [unwired: 1 in]
            n191 = Insert Into Array(array=w450, new element=w445) -> (w448:cluster{"ThreadName":string, "Fail":bool}[])  [unwired: 1 in]
          }
        }
        n192 = Bundle By Name(cluster=w424, "FailedThreads"=w412, "Error"=w415, "Threads.Cfg"=w410) -> (w423:T5)
      }
      frame "Oper :Call SavePara UI" {
        w453 = FALSE ("open front panel? (T)")
        n193 = vi-ref "Save Para Setting UI.vi"() -> (w452:refnum<vi>)
        n194 = Unbundle By Name(w465) -> ("FailedThreads"=w458:cluster{"ThreadName":string, "Fail":bool}[], "Error"=w467:errorcluster, "LocalQ.LocalName"=w451:string, "InsertUI"=w463:string)
        n195 = property class="VI"(reference=w452, error in=w467) -> (reference out=w456:refnum<vi>, error out=w468:errorcluster, "Name"=w455:string, "Path"=w466:path)
        n196 = call "ARC_Dynamic Call_Single.vi"("command queue name"=w455, "open front panel? (T)"=w453, "error in (no error)"=w468, "parameter else"=w451, "control name"="Parameter", "vi path"=w466) -> ("error out"=w461:errorcluster, "call failed"=w459:bool)  [unwired: 3 in, 1 out]
        n197 = Equal?(x="SavePara" ("control name"), y=w463) -> (x = y?=w454:bool)
        n198 = case shown="False" w459 {
          selector: w459 -> [_ w490]
          tunnel: w461 -> [w474 w488]
          tunnel: w458 -> [w476 w491]
          tunnel: [w476 w489] -> w457
          tunnel: [w475 w488] -> w460
          tunnel: w454 -> [w473 _]
          tunnel: w456 -> [w472 _]
          tunnel: w455 -> [_ w487]
          tunnel: w453 -> [w471 _]
          frame False {
            n199 = case shown="True" w473 {
              tunnel: [w477 w481] -> w475
              tunnel: w472 -> [_ w480]
              tunnel: w474 -> [w477 w479]
              tunnel: w471 -> [_ w478]
              frame False {
              }
              frame True {
                n200 = case shown="False" w478 {
                  tunnel: [w484 w485] -> w481
                  tunnel: w480 -> [w483 _]
                  tunnel: w479 -> [w482 w485]
                  frame False {
                    n201 = invoke on="子面板" class="SubPnl" method="Insert VI"(error in=w482, "VI Ref"=w483) -> (error out=w484:errorcluster)  [unwired: 2 in, 3 out]
                  }
                  frame True {
                  }
                }
              }
            }
          }
          frame True {
            n202 = Bundle("Name"=w487, w490) -> (w486:cluster{"Name":string, bool})  [unwired: 1 in]
            n203 = Insert Into Array(array=w491, new element=w486) -> (w489:cluster{"ThreadName":string, "Fail":bool}[])  [unwired: 1 in]
          }
        }
        n204 = Bundle By Name(cluster=w465, "FailedThreads"=w457, "Error"=w460, "Threads.SavePara"=w455) -> (w464:T5)
      }
      frame "Oper :Call Display Graph" {
        w493 = "Q_Disp" ("y")
        w492 = FALSE ("open front panel? (T)")
        n205 = vi-ref "Graph and List Display UI.vi"() -> (w504:refnum<vi>)
        n206 = Unbundle By Name(w506) -> ("FailedThreads"=w502:cluster{"ThreadName":string, "Fail":bool}[], "Error"=w508:errorcluster, "LocalQ.LocalName"=w498:string, "InsertUI"=w497:string)
        n207 = property class="VI"(reference=w504, error in=w508) -> (reference out=w494:refnum<vi>, error out=w509:errorcluster, "Name"=w501:string, "Path"=w507:path)
        n208 = call "ARC_Dynamic Call_Single.vi"("command queue name"=w493, "open front panel? (T)"=w492, "error in (no error)"=w509, "parameter else"=w498, "control name"="Parameter", "vi path"=w507) -> ("error out"=w503:errorcluster, "call failed"=w496:bool)  [unwired: 3 in, 1 out]
        n209 = Equal?(x=w493, y=w497) -> (x = y?=w495:bool)
        n210 = case shown="False" w496 {
          selector: w496 -> [_ w530]
          tunnel: w503 -> [w515 w527]
          tunnel: w502 -> [w517 w532]
          tunnel: w501 -> [_ w531]
          tunnel: [w517 w528] -> w500
          tunnel: [w514 w527] -> w499
          tunnel: w495 -> [w516 _]
          tunnel: w494 -> [w513 _]
          tunnel: w492 -> [w512 _]
          frame False {
            n211 = case shown="True" w516 {
              tunnel: w515 -> [w518 w522]
              tunnel: [w518 w521] -> w514
              tunnel: w513 -> [_ w520]
              tunnel: w512 -> [_ w519]
              frame False {
              }
              frame True {
                n212 = case shown="False" w519 {
                  tunnel: w522 -> [w525 w526]
                  tunnel: [w524 w526] -> w521
                  tunnel: w520 -> [w523 _]
                  frame False {
                    n213 = invoke on="子面板" class="SubPnl" method="Insert VI"(error in=w525, "VI Ref"=w523) -> (error out=w524:errorcluster)  [unwired: 2 in, 3 out]
                  }
                  frame True {
                  }
                }
              }
            }
          }
          frame True {
            n214 = Bundle("Name"=w531, w530) -> (w529:cluster{"Name":string, bool})  [unwired: 1 in]
            n215 = Insert Into Array(array=w532, new element=w529) -> (w528:cluster{"ThreadName":string, "Fail":bool}[])  [unwired: 1 in]
          }
        }
        n216 = Bundle By Name(cluster=w506, "FailedThreads"=w500, "Error"=w499, "Threads.Disp"=w493) -> (w505:T5)
      }
      frame "Oper :Call Data Thread" {
        w536 = "Q_Data" ("y")
        n217 = Unbundle By Name(w547) -> ("FailedThreads"=w543:cluster{"ThreadName":string, "Fail":bool}[], "Error"=w549:errorcluster, "LocalQ.LocalName"=w539:string, "Buffers.DataBuf"=w533:refnum<queue>)
        n218 = vi-ref "Data Thread.vi"() -> (w545:refnum<vi>)
        n219 = property class="VI"(reference=w545, error in=w549) -> (reference out=w537:refnum<vi>, error out=w550:errorcluster, "Name"=w542:string, "Path"=w548:path)
        n220 = Bundle("LocalName"=w539, "DataBuf"=w533) -> (w534:T12)  [unwired: 1 in]
        n221 = call "ARC_Dynamic Call_Single.vi"("command queue name"=w536, "open front panel? (T)"=FALSE, "error in (no error)"=w550, "parameter else"=w534, "control name"="Parameter", "vi path"=w548) -> ("error out"=w544:errorcluster, "call failed"=w538:bool)  [unwired: 3 in, 1 out]
        n222 = case shown="True" w538 {
          selector: w538 -> [_ w558]
          tunnel: w544 -> [w553 w555]
          tunnel: w543 -> [w554 w560]
          tunnel: w542 -> [_ w559]
          tunnel: [w554 w556] -> w541
          tunnel: [w553 w555] -> w540
          tunnel: w537 -> [_ _]
          frame False {
          }
          frame True {
            n223 = Bundle("Name"=w559, w558) -> (w557:cluster{"Name":string, bool})  [unwired: 1 in]
            n224 = Insert Into Array(array=w560, new element=w557) -> (w556:cluster{"ThreadName":string, "Fail":bool}[])  [unwired: 1 in]
          }
        }
        n225 = Bundle By Name(cluster=w547, "FailedThreads"=w541, "Error"=w540, "Threads.Data"=w536) -> (w546:T5)
      }
      frame "Oper :Call Welcome UI" {
        n226 = Unbundle By Name(w576) -> ("FailedThreads"=w569:cluster{"ThreadName":string, "Fail":bool}[], "Error"=w578:errorcluster, "LocalQ.LocalName"=w574:string, "Path.System Config"=w572:path, "InsertUI"=w563:string)
        n227 = vi-ref "Welcome UI.vi"() -> (w567:refnum<vi>)
        n228 = property class="VI"(reference=w567, error in=w578) -> (error out=w579:errorcluster, "Name"=w564:string, "Path"=w577:path)  [unwired: 1 out]
        n229 = Equal?(x=w563, y="Welcome UI") -> (x = y?=w562:bool)
        n230 = Bundle("LocalName"=w574, "System Config"=w572) -> (w573:T13)  [unwired: 1 in]
        n231 = call "ARC_Dynamic Call_Single.vi"("command queue name"=w564, "open front panel? (T)"=FALSE, "error in (no error)"=w579, "parameter else"=w573, "control name"="Parameter", "vi path"=w577) -> ("error out"=w571:errorcluster, "time out"=w581:bool, "call failed"=w565:bool)  [unwired: 3 in]
        n232 = Compound Arithmetic op=OR(invert w565, invert w581, w562) -> (w566:bool)
        n233 = case shown="False" w565 {
          selector: w565 -> [_ w596]
          tunnel: w571 -> [w586 w593]
          tunnel: w569 -> [w588 w598]
          tunnel: w564 -> [_ w597]
          tunnel: [w588 w594] -> w568
          tunnel: [w587 w593] -> w570
          tunnel: w566 -> [w585 _]
          tunnel: w567 -> [w584 _]
          frame False {
            n234 = case shown="False" w585 {
              tunnel: [w589 w592] -> w587
              tunnel: w584 -> [_ w591]
              tunnel: w586 -> [w589 w590]
              frame False {
              }
              frame True {
                n235 = invoke on="子面板" class="SubPnl" method="Insert VI"(error in=w590, "VI Ref"=w591) -> (error out=w592:errorcluster)  [unwired: 2 in, 3 out]
              }
            }
          }
          frame True {
            n236 = Bundle("Name"=w597, w596) -> (w595:cluster{"Name":string, bool})  [unwired: 1 in]
            n237 = Insert Into Array(array=w598, new element=w595) -> (w594:cluster{"ThreadName":string, "Fail":bool}[])  [unwired: 1 in]
          }
        }
        n238 = Bundle By Name(cluster=w576, "FailedThreads"=w568, "Error"=w570) -> (w575:T5)
      }
      frame "Oper :Call OPC Read Bool UI" {
        n239 = Unbundle By Name(w604) -> ("Error"=w606:errorcluster, "LocalQ.LocalName"=w602:string)
        n240 = vi-ref "OPC Read Bool Variables.vi"() -> (w599:refnum<vi>)
        n241 = property class="VI" props=["Name", "Path"](reference=w599, error in=w606) -> (error out=w607:errorcluster, "Path"=w605:path)  [unwired: 2 out]
        n242 = call "ARC_Dynamic Load.vi"("Auto Dispose Ref"=FALSE ("open front panel? (T)"), "error in"=w607, "CtrlValue"=w602, "CtrlName"="Caller" ("control name"), "Vi Path"=w605) -> ("错误输出"=w601:errorcluster)  [unwired: 5 in, 1 out]
        n243 = invoke on="toppanel" class="SubPnl" method="Insert VI"(error in=w601, "VI Ref"=w599) -> (error out=w600:errorcluster)  [unwired: 2 in, 3 out]
        n244 = Bundle By Name(cluster=w604, "Error"=w600) -> (w603:T5)
      }
      frame "Oper :Call DAQ Mean Data UI" {
        w611 = FALSE ("open front panel? (T)")
        n245 = Unbundle By Name(w617) -> ("Error"=w619:errorcluster, "LocalQ.LocalName"=w615:string)
        n246 = vi-ref "DAQ Mean Data UI.vi"() -> (w612:refnum<vi>)
        n247 = property class="VI" props=["Name", "Path"](reference=w612, error in=w619) -> (error out=w620:errorcluster, "Path"=w618:path)  [unwired: 2 out]
        n248 = call "ARC_Dynamic Load.vi"("Auto Dispose Ref"=w611, "error in"=w620, "CtrlValue"=w615, "CtrlName"="Caller" ("control name"), "Vi Path"=w618) -> ("错误输出"=w614:errorcluster)  [unwired: 5 in, 1 out]
        n249 = case shown="False" w611 {
          tunnel: w614 -> [w625 w626]
          tunnel: [w624 w626] -> w613
          tunnel: w612 -> [w623 _]
          frame False {
            n250 = invoke on="botmPanel" class="SubPnl" method="Insert VI"(error in=w625, "VI Ref"=w623) -> (error out=w624:errorcluster)  [unwired: 2 in, 3 out]
          }
          frame True {
          }
        }
        n251 = Bundle By Name(cluster=w617, "Error"=w613) -> (w616:T5)
      }
      frame "Oper :Call User WorkTable-1#" {
        n252 = disable-structure shown="Disabled" {
          disable-tunnel: w628 -> [w639 w649]
          disable-tunnel: [w638 w649] -> w627
          frame Disabled {
            n253 = Unbundle By Name(w639) -> ("Error"=w641:errorcluster, "LocalQ.LocalName"=w637:string, "InsertUI"=w632:string)
            n254 = vi-ref "UserWorkTable-1#.vi"() -> (w636:refnum<vi>)
            n255 = property class="VI" props=["Name", "Path"](reference=w636, error in=w641) -> (error out=w642:errorcluster, "Path"=w640:path)  [unwired: 2 out]
            n256 = Equal?(x=w632, y="UserWorkTable-1#") -> (x = y?=w630:bool)
            n257 = call "ARC_Dynamic Load.vi"("Auto Dispose Ref"=FALSE ("open front panel? (T)"), "error in"=w642, "CtrlValue"=w637, "CtrlName"="Caller" ("control name"), "Vi Path"=w640) -> ("错误输出"=w635:errorcluster, "vi reference"=w633:refnum<vi>)  [unwired: 5 in]
            n258 = case shown="True" w630 {
              tunnel: w635 -> [w645 w648]
              tunnel: [w645 w647] -> w634
              tunnel: w633 -> [_ w646]
              frame False {
              }
              frame True {
                n259 = invoke on="子面板" class="SubPnl" method="Insert VI"(error in=w648, "VI Ref"=w646) -> (error out=w647:errorcluster)  [unwired: 2 in, 3 out]
              }
            }
            n260 = Bundle By Name(cluster=w639, "Error"=w634) -> (w638:T5)
          }
          frame Enabled {
          }
        }
      }
      frame "Oper :Call Error Handle" {
        n261 = Unbundle By Name(w659) -> ("FailedThreads"=w652:cluster{"ThreadName":string, "Fail":bool}[], "Error"=w661:errorcluster, "LocalQ.LocalName"=w656:string)
        n262 = vi-ref "Error Handle.vi"() -> (w657:refnum<vi>)
        n263 = property class="VI"(reference=w657, error in=w661) -> (error out=w662:errorcluster, "Name"=w650:string, "Path"=w660:path)  [unwired: 1 out]
        n264 = call "ARC_Dynamic Call_Single.vi"("command queue name"=w650, "open front panel? (T)"=FALSE, "error in (no error)"=w662, "parameter else"=w656, "control name"="Parameter", "vi path"=w660) -> ("error out"=w655:errorcluster, "call failed"=w654:bool)  [unwired: 3 in, 1 out]
        n265 = case shown="True" w654 {
          selector: w654 -> [_ w671]
          tunnel: w655 -> [w667 w668]
          tunnel: w652 -> [w666 w673]
          tunnel: w650 -> [_ w672]
          tunnel: [w666 w669] -> w651
          tunnel: [w667 w668] -> w653
          frame False {
          }
          frame True {
            n266 = Bundle("Name"=w672, w671) -> (w670:cluster{"Name":string, bool})  [unwired: 1 in]
            n267 = Insert Into Array(array=w673, new element=w670) -> (w669:cluster{"ThreadName":string, "Fail":bool}[])  [unwired: 1 in]
          }
        }
        n268 = Bundle By Name(cluster=w659, "FailedThreads"=w651, "Error"=w653) -> (w658:T5)
      }
      frame "Oper :Thread Loaded Fail" {
        n269 = Unbundle By Name(w681) -> ("FailedThreads"=w679:cluster{"ThreadName":string, "Fail":bool}[], "Error"=w680:errorcluster)
        n270 = Empty Array?(array=w679) -> (empty?=w678:bool)
        n271 = case shown="True" w678 {
          tunnel: w679 -> [w688 _]
          tunnel: w680 -> [w687 w690]
          tunnel: [w684 w689] -> w674
          tunnel: ["UI :L_Core - Exit System" ("Error Handle") _] -> w676
          frame False {
            n272 = call "GEN_Load Fail Clue Info.vi"("error in (no error)"=w687, "Failed LoadedT"=w688) -> ("error out"=w686:errorcluster, "User Clue out"=w685:string)  [unwired: 8 in]
            n273 = call "GEN_Double Buttons ClueWindow.vi"("error in (no error)"=w686, "Content Input"=w685) -> ("error out"=w684:errorcluster)  [unwired: 7 in, 2 out]
          }
          frame True {
            n274 = call "GEN_State Notifier.vi"("Action Select"=T2."Send Notification", "error in (no error)"=w690, "Notification"="") -> ("error out"=w689:errorcluster)  [unwired: 7 in, 1 out]
          }
        }
        n275 = Build Array (concatenate)(w676, w682) -> (w677:string[])
        n276 = Bundle By Name(cluster=w681, "Error"=w674) -> (w675:T5)
      }
      frame "//Oper :Set Splitter Position" {
        n277 = Unbundle By Name(w702) -> ("InsertUI"=w701:string, "Error"=w700:errorcluster)
        n278 = property class="VI"(error in=w700) -> (error out=w699:errorcluster, "Front Panel.PanelBounds"=w698:T14)  [unwired: 1 in, 1 out]
        n279 = Unbundle By Name(w698) -> ("Bottom"=w693:i16, "Top"=w697:i16)
        n280 = Subtract(x=w693, y=w697) -> (x-y=w696:i16)
        n281 = case shown="Default" w701 {
          tunnel: w699 -> [w712 w720]
          tunnel: [w711 w718] -> w694
          tunnel: w696 -> [w709 w716]
          tunnel: w693 -> [w706 _]
          frame Default {
            n282 = Multiply(x=0.1, y=w709) -> ()  [unwired: 1 out]
            n283 = property on="分隔栏 4" class="Splitter"(error in=w712, "Position"=70 ("分隔栏位置")) -> (error out=w713:errorcluster)  [unwired: 1 in, 1 out]
            n284 = Multiply(x=0.3, y=w709) -> (x*y=w707:dbl)
            n285 = Subtract(x=w706, y=w707) -> ()  [unwired: 1 out]
            n286 = property on="分隔栏 5" class="Splitter"(error in=w713, "Position"=850 ("分隔栏位置")) -> (error out=w711:errorcluster)  [unwired: 1 in, 1 out]
          }
          frame "", "Device", "SavePara" {
            # "隐藏上下两个子面板"
            n287 = Subtract(x=w716, y=i16 13) -> (x-y=w714:i16)
            n288 = property on="分隔栏 4" class="Splitter"(error in=w720, "Position"=12 ("分隔栏位置")) -> (error out=w719:errorcluster)  [unwired: 1 in, 1 out]
            n289 = property on="分隔栏 5" class="Splitter"(error in=w719, "Position"=w714) -> (error out=w718:errorcluster)  [unwired: 1 in, 1 out]
          }
        }
        n290 = Bundle By Name(cluster=w702, "Error"=w694) -> (w695:T5)
      }
      frame "Oper :Tree - Initialize" {
        n291 = Unbundle By Name(w725) -> ("Ref.Tree"=w721:refnum<vi>, "Error"=w723:errorcluster)
        n292 = call "Main Tree _ Initialize.vi"("error in"=w723, "Ref.Tree Ref"=w721) -> ("error out"=w722:errorcluster)  [unwired: 9 in]
        n293 = Bundle By Name(cluster=w725, "Error"=w722) -> (w724:T5)
      }
      frame "Oper :Tree - Add VCH" {
        n294 = Unbundle By Name(w731) -> ("Ref.Tree"=w729:refnum<vi>, "Error"=w728:errorcluster)
        n295 = call "Main Tree _ Add VCH Tag.vi"("error in"=w728, "Ref.Tree Ref"=w729) -> ("error out"=w727:errorcluster)  [unwired: 9 in]
        n296 = Bundle By Name(cluster=w731, "Error"=w727) -> (w730:T5)
      }
      frame "UI :L_Oper - Defer FP Update" {
        n297 = Unbundle By Name(w735) -> ("Ref.VIRef"=w741:refnum<vi>, "Error"=w742:errorcluster)
        n298 = property class="VI"(reference=w741, error in=w742) -> (error out=w740:errorcluster, "Panel"=w739:refnum<vi>)  [unwired: 1 out]
        n299 = property class="Pnl"(reference=w739, error in=w740, "DeferPanUpdts"=TRUE ("延迟前面板更新")) -> (reference out=w737:refnum<vi>, error out=w738:errorcluster)
        n300 = Close Reference(reference=w737, error in (no error)=w738) -> (error out=w736:errorcluster)
        n301 = Bundle By Name(cluster=w735, "Error"=w736) -> (w734:T5)
      }
      frame "UI :L_Oper - FP Update" {
        n302 = Unbundle By Name(w746) -> ("Ref.VIRef"=w752:refnum<vi>, "Error"=w753:errorcluster)
        n303 = property class="VI"(reference=w752, error in=w753) -> (error out=w751:errorcluster, "Panel"=w750:refnum<vi>)  [unwired: 1 out]
        n304 = property class="Pnl"(reference=w750, error in=w751, "DeferPanUpdts"=FALSE ("延迟前面板更新")) -> (reference out=w748:refnum<vi>, error out=w749:errorcluster)
        n305 = Close Reference(reference=w748, error in (no error)=w749) -> (error out=w747:errorcluster)
        n306 = Bundle By Name(cluster=w746, "Error"=w747) -> (w745:T5)
      }
      frame "UI :L_Oper - Set Mouse Busy" {
        n307 = Unbundle By Name(w757) -> ("Ref.VIRef"=w756:refnum<vi>)
        n308 = call <vilib>:"Set Busy.vi"("disable click? (T)"=FALSE, "VI reference (current VI)"=w756) -> ()  [unwired: 8 in, 2 out]
      }
      frame "UI :L_Oper - Set Mouse Free" {
        n309 = Unbundle By Name(w759) -> ("Ref.VIRef"=w760:refnum<vi>)
        n310 = call <vilib>:"Unset Busy.vi"("VI reference (current VI)"=w760) -> ()  [unwired: 10 in, 1 out]
      }
      frame "UI :L_Oper - Initialize Tree Custom Symbol" {
        n311 = Unbundle By Name(w770) -> ("Path.System Config"=w765:path, "Ref.Tree"=w769:refnum<vi>, "Error"=w768:errorcluster)
        n312 = Strip Path(path=w765) -> (stripped path=w764:path)  [unwired: 1 out]
        n313 = Build Path(base path=w764, name or relative path="Tree PNG") -> (appended path=w762:path)
        n314 = call "TREE_List Symbol Custom.vi"("error in"=w768, "PicturePath"=w762, "ListRef"=w769) -> ("error out"=w766:errorcluster)  [unwired: 7 in, 1 out]
        n315 = Bundle By Name(cluster=w770, "Error"=w766) -> (w767:T5)
      }
      frame "Oper :Scan for Devices" {
        w773 = "Gantner" ("DevName")
        # "获取当前系统中的硬件信息；\n硬件列表刷新至前面板树控件；"
        n316 = Unbundle By Name(w782) -> ("Ref.Tree"=w775:refnum<vi>, "Error"=w781:errorcluster)
        n317 = call "HW_Gantner_DAQ FGV.vi"("DevName"=w773, "Oper."=DAQ_FGV_Operations."Search", "error in"=w781) -> ("Cfg out"=w772:T15[], "error out"=w777:errorcluster)  [unwired: 6 in, 5 out]
        n318 = call "HW_Gantner_Refresh Tree Device Info.vi"("Cfg"=w772, "error in"=w777, "Device"=w773, "Ref.Tree Ref"=w775) -> ("error out"=w776:errorcluster)  [unwired: 7 in]
        n319 = Build Array (concatenate)(string[] ["Oper :Get First Module", "Event :Main-->Cfg - Start DAQ"] ("event queue out"), w783) -> (w779:string[])
        n320 = Bundle By Name(cluster=w782, "DevName"=w773, "Error"=w776) -> (w780:T5)
      }
      frame "Oper :Get First Module" {
        n321 = Unbundle By Name(w790) -> ("Ref.Tree"=w788:refnum<vi>, "Error"=w789:errorcluster)
        n322 = call "TREE_Get First Child Only Tag.vi"("error in"=w789, "Parent Tag"="Device", "Tree Ref"=w788) -> ("error out"=w785:errorcluster, "tag out"=w784:string)  [unwired: 7 in]
        n323 = Bundle By Name(cluster=w790, "LocalQ.LocalData"=w784, "Error"=w785) -> (w786:T5)
      }
      frame "Oper :Create Buffers" {
        n324 = Unbundle By Name(w799) -> ("Error"=w798:errorcluster)
        n325 = Obtain Queue(max queue size (-1, unlimited)=100, name (unnamed)="Data", element data type=waveform(dbl)[] [] ("data"), error in (no error)=w798) -> (queue out=w792:refnum<queue>, error out=w793:errorcluster)  [unwired: 1 in, 1 out]
        n326 = Bundle By Name(cluster=w799, "Buffers.DataBuf"=w792, "Error"=w793) -> (w794:T5)
      }
      frame "----------Communication----------" {
      }
      frame "Oper :Send To LowLevel" {
        n327 = Unbundle By Name(w803) -> ("Q-LowLevel.Q-LowLevel Name"=w805:string, "Q-LowLevel.Q-LowLevel Order"=w808:string, "Q-LowLevel.Q-LowLevel Data"=w809:variant, "Error"=w806:errorcluster)
        n328 = call-poly "ARC_Queue Management.vi"("Queue Name(unamed)"=w805) -> ("Not Exist?"=w807:bool)  [unwired: 8 in, 2 out]
        n329 = case shown="False" w807 {
          tunnel: w806 -> [w817 w818]
          tunnel: w805 -> [w815 _]
          tunnel: w808 -> [w813 _]
          tunnel: w809 -> [w814 _]
          tunnel: [w812 w818] -> w804
          frame False {
            n330 = call-poly "ARC_Queue Management.vi"("Time out(-1)_queue in"=50, "error in (no error)"=w817, "Data"=w814, "Event"=w813, "Queue Name(unamed)"=w815) -> ("error out"=w812:errorcluster)  [unwired: 5 in, 1 out]
          }
          frame True {
          }
        }
        n331 = Bundle By Name(cluster=w803, "Error"=w804) -> (w810:T5)
      }
    }
    n332 = Unbundle By Name(w131) -> ("Exit"=w130:bool)
  }
  n333 = Unbundle By Name(w17) -> ("Ref.VIRef"=w23:refnum<vi>, "LocalQ.LocalName"=w19:string, "Error"=w18:errorcluster)
  n334 = disable-structure shown="禁用" {
    frame Disabled {
    }
    frame Enabled {
    }
  }
  n335 = call-poly "ARC_Queue Management.vi"("error in (no error)"=w18, "Queue Name(unamed)"=w19) -> ("error out"=w22:errorcluster)  [unwired: 7 in, 2 out]
  n336 = call "ARC_Comm Application Exit.vi"("error in (no error)"=w22, "This VI"=w23) -> ()  [unwired: 9 in, 1 out]
